vi "select ROIS.vi"(8 "error in (no error)":errorcluster, 11 "Cascade in":refnum<class "Cascade.lvclass">) -> (0 "error out":errorcluster, 3 "Cascade out":refnum<class "Cascade.lvclass">)   [LabVIEW 2012, in "Cascade.lvclass"]
uses:
  Cascade.lvclass
  Cascade.lvclass/Cascade.ctl
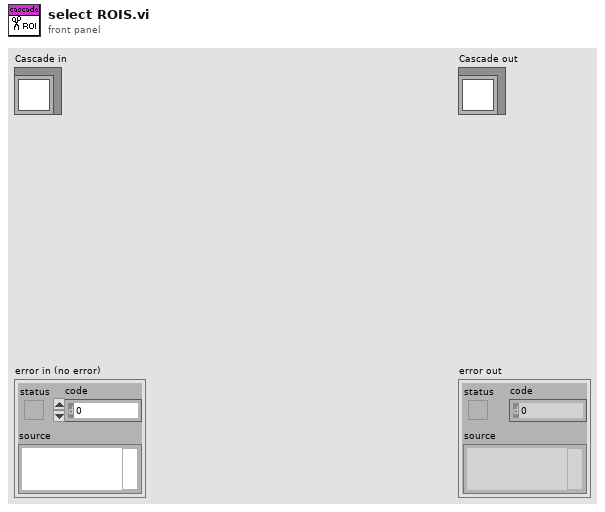
[diagram p1: front panel]
types:
  T1 = typedef "IMAQ Image.ctl" = refnum<image>
  T2 = typedef "ROI Descriptor" = cluster{"Global Rectangle":i32[], "Contours":cluster{"ID":enum32{"External", "Internal"}, "Type":u32, "Coordinates":i32[]}[]}
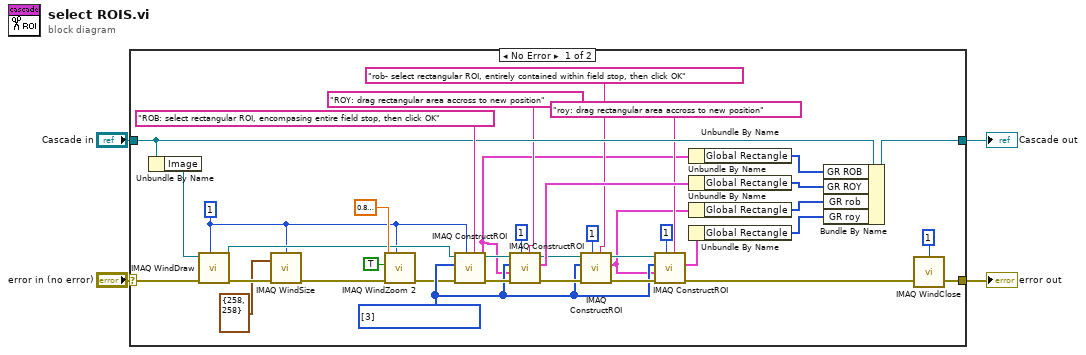
[diagram p0: block diagram]
diagram:
  n1 = case shown="No Error" "error in (no error)" {
    selector: "error in (no error)" -> [w37 w43]
    tunnel: [w22 w43] -> w3
    tunnel: [w19 w42] -> w1
    tunnel: "Cascade in" -> [w20 w42]
    frame No Error {
      w6 = 1 ("Window Number (0...15)")
      w25 = u32[] [3] items=["No Selection", "Point", "Line", "Rectangle", "Oval", "Polygon", "Freehand Region", "Annulus", "Zoom", "Pan", "Broken Line", "Freehand Line", "Rotated Rectangle"] ("Tools")
      n2 = Unbundle By Name(w20) -> ("Image"=w38:T1)
      n3 = call "IMAQ WindDraw"("Window Number (0...15)"=w6, "error in (no error)"=w37, "Image"=w38) -> ("error out"=w8:errorcluster, "Image Out (duplicate)"=w40:T1)  [unwired: 7 in]
      n4 = call "IMAQ WindSize"("error in (no error)"=w8, "Width & Height"=cluster{"Width":i32, "Height":i32} {"Width"=258, "Height"=258}, "Window Number"=w6) -> ("error out"=w7:errorcluster)  [unwired: 3 in, 2 out]
      n5 = call "IMAQ WindZoom 2"("Window Number (0...15)"=w6, "error in (no error)"=w7, "Zoom to Fit? (False)"=TRUE, "Zoom Factor"=sgl 0.9) -> ("error out"=w9:errorcluster)  [unwired: 4 in, 3 out]
      n6 = call "IMAQ ConstructROI"("Prompt"="ROB: select rectangular ROI, encompasing entire field stop, then click OK", "Window Number (-1...15)"=w6, "error in (no error)"=w9, "Tools"=w25, "Image"=w40) -> ("error out"=w34:errorcluster, "ROI Descriptor Out"=w11:T2, "Image Out (duplicate)"=w33:T1)  [unwired: 3 in, 1 out]
      n7 = call "IMAQ ConstructROI"("Prompt"="ROY: drag rectangular area accross to new position", "Window Number (-1...15)"=1, "error in (no error)"=w34, "ROI Descriptor In (None)"=w11, "Tools"=w25, "Image"=w33) -> ("error out"=w29:errorcluster, "ROI Descriptor Out"=w32:T2, "Image Out (duplicate)"=w27:T1)  [unwired: 2 in, 1 out]
      n8 = call "IMAQ ConstructROI"("Prompt"="rob- select rectangular ROI, entirely contained within field stop, then click OK", "Window Number (-1...15)"=1, "error in (no error)"=w29, "Tools"=w25, "Image"=w27) -> ("error out"=w28:errorcluster, "ROI Descriptor Out"=w10:T2, "Image Out (duplicate)"=w26:T1)  [unwired: 3 in, 1 out]
      n9 = call "IMAQ ConstructROI"("Prompt"="roy: drag rectangular area accross to new position", "Window Number (-1...15)"=1, "error in (no error)"=w28, "ROI Descriptor In (None)"=w10, "Tools"=w25, "Image"=w26) -> ("error out"=w21:errorcluster, "ROI Descriptor Out"=w24:T2)  [unwired: 2 in, 2 out]
      n10 = Unbundle By Name(w11) -> ("Global Rectangle"=w18:i32[])
      n11 = Unbundle By Name(w32) -> ("Global Rectangle"=w17:i32[])
      n12 = Unbundle By Name(w10) -> ("Global Rectangle"=w16:i32[])
      n13 = Unbundle By Name(w24) -> ("Global Rectangle"=w15:i32[])
      n14 = Bundle By Name(cluster=w20, "GR ROB"=w18, "GR ROY"=w17, "GR rob"=w16, "GR roy"=w15) -> (w19:refnum<class "Cascade.lvclass">)
      n15 = call "IMAQ WindClose"("Window Number (0...15)"=1, "error in (no error)"=w21) -> ("error out"=w22:errorcluster)  [unwired: 4 in]
    }
    frame Error {
    }
  }
  "error out" <- w3
  "Cascade out" <- w1
